vi "UpdateSetTerm.vi"(2 "State In":T1 {"BlockNodeState"."Draw Style" items=["FunctionBlock", "ExpressVI", "Variable", "Elemental I/O", "32x32 Icon", "FunctionBlockCompact"]; "BlockNodeState"."Terminal Data"."Terminal Flags" format="%.0b"}) -> (0 "State Out":T1 {"BlockNodeState"."Draw Style" items=["FunctionBlock", "ExpressVI", "Variable", "Elemental I/O", "32x32 Icon", "FunctionBlockCompact"]; "BlockNodeState"."Terminal Data"."Terminal Flags" format="%.0b"})   [LabVIEW 2017, in "Set DDT Attributes.lvlib"]
uses:
  <vilib>/express/express signal manip/GetorSetDDTAttributes/Set DDT Attributes/Set DDT Attributes.lvlib
  <vilib>/express/express signal manip/GetorSetDDTAttributes/Set DDT Attributes/State.ctl
  <vilib>/BlockNodeSupport/BlockNodeState.ctl
  <vilib>/BlockNodeSupport/TerminalData.ctl
  <vilib>/picture/picture.llb/imagedata.ctl
  <vilib>/express/express signal manip/GetorSetDDTAttributes/Shared VIs/Attributes data.ctl
  <vilib>/express/express signal manip/GetorSetDDTAttributes/Shared VIs/Input.ctl
  <vilib>/express/express signal manip/GetorSetDDTAttributes/Shared VIs/Attributes name.ctl
  <vilib>/express/express signal manip/GetorSetDDTAttributes/Shared VIs/GetSetShared.lvlib
  <vilib>/express/express signal manip/GetorSetDDTAttributes/Set DDT Attributes/Set DDT Properties.xnode
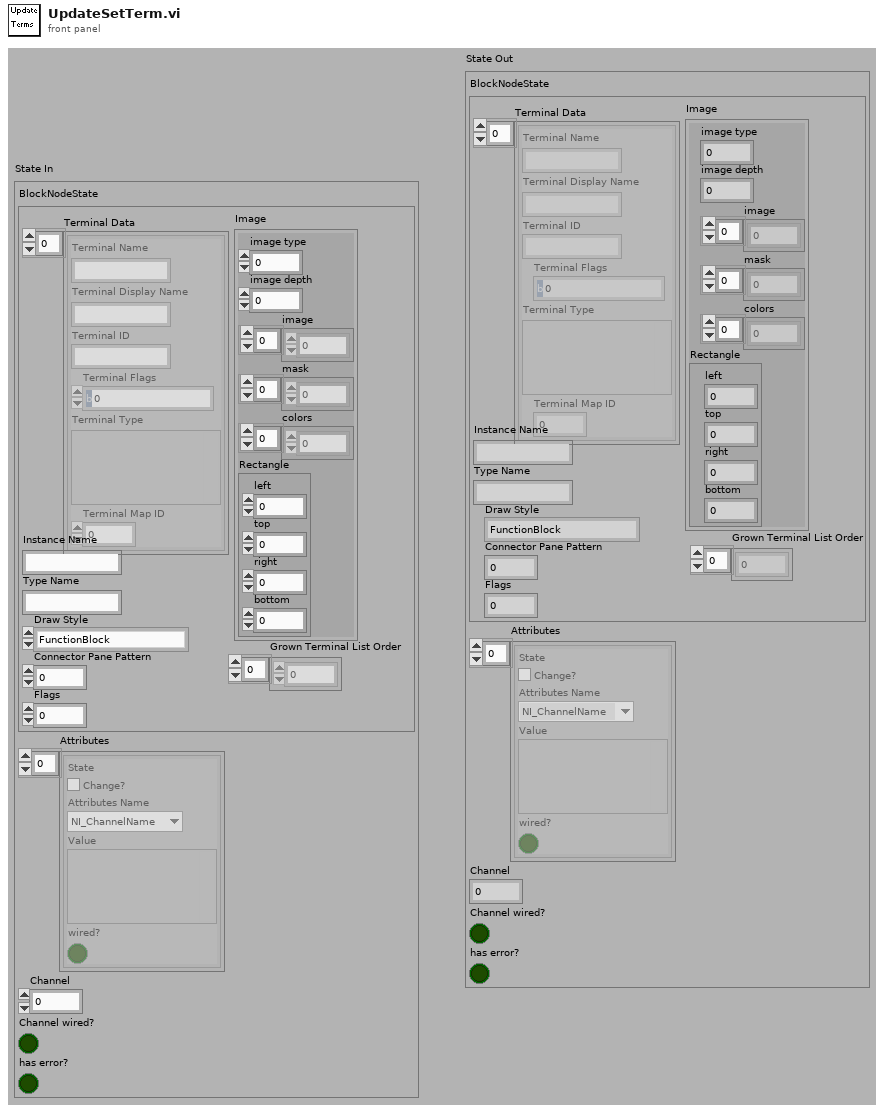
[diagram p1: front panel]
types:
  T1 = typedef "Set DDT Attributes.lvlib/Set DDT Properties.xnode/State.ctl" = cluster{"BlockNodeState":T2, "Attributes":T5[], "Channel":u32, "Channel wired?":bool, "has error?":bool}
  T2 = typedef "BlockNodeState.ctl" = cluster{"Terminal Data":T3[], "Instance Name":string, "Type Name":string, "Draw Style":i32, "Connector Pane Pattern":i32, "Flags":i32, "Grown Terminal List Order":i32[], "Image":T4}
  T3 = typedef "TerminalData.ctl" = cluster{"Terminal Name":string, "Terminal Display Name":string, "Terminal ID":string, "Terminal Flags":i32, "Terminal Type":variant, "Terminal Map ID":i32}
  T4 = typedef "imagedata.ctl" = cluster{"image type":i32, "image depth":i32, "image":u8[], "mask":u8[], "colors":u32[], "Rectangle":cluster{"left":i16, "top":i16, "right":i16, "bottom":i16}}
  T5 = typedef "GetSetShared.lvlib/Attributes data.ctl" = cluster{"State":T6, "Attributes Name":T7, "Value":variant, "wired?":bool}
  T6 = typedef "GetSetShared.lvlib/Input.ctl" = bool
  T7 = typedef "GetSetShared.lvlib/Attributes name.ctl" = enum16{"NI_ChannelName", "NI_ExpIsRelativeTime", "NI_ExpTimeStamp", "NI_ExpStartTimeStamp", "NI_ExpXDimension", "NI_UnitDescription"}
  T8 = cluster{"Terminal Name":string, "Terminal Display Name":string, "Terminal ID":string, "Terminal Flags":i32, "Terminal Type":variant, "Terminal Map ID":i32}
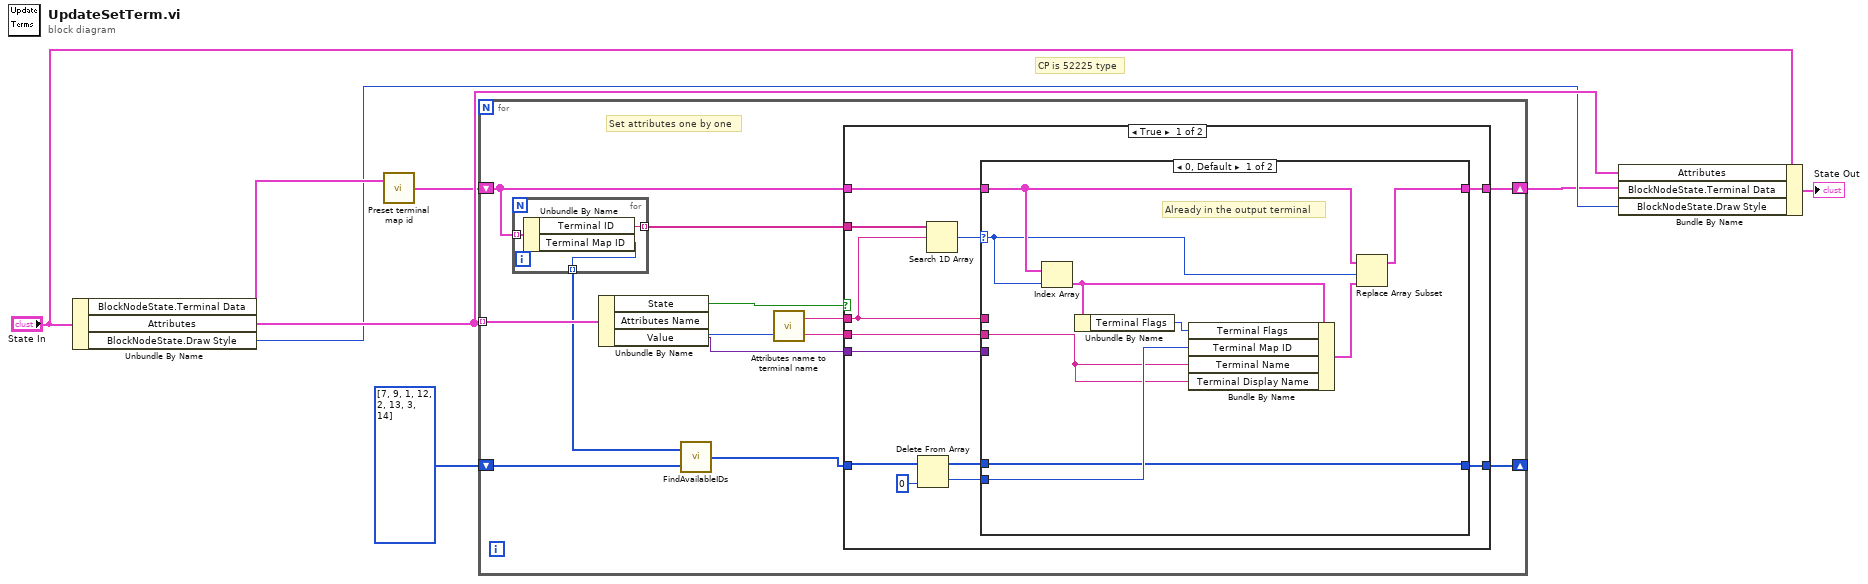
[diagram p0: block diagram]
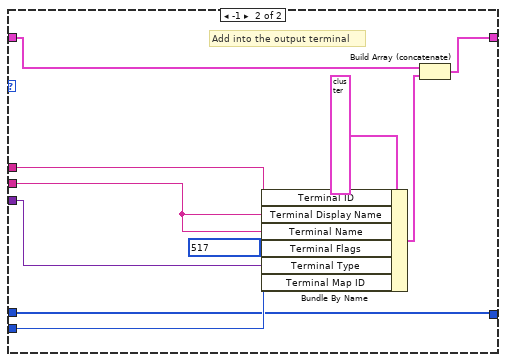
[diagram p2: hidden frame]
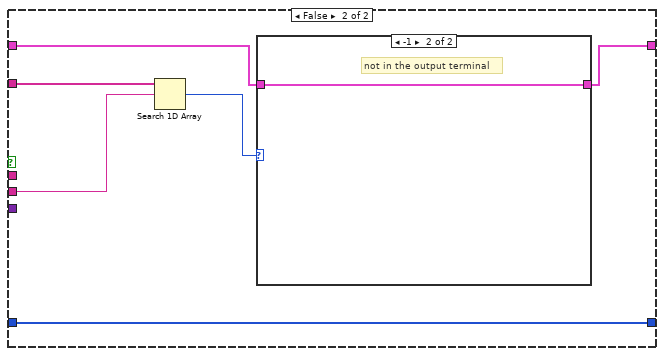
[diagram p3: hidden frame]
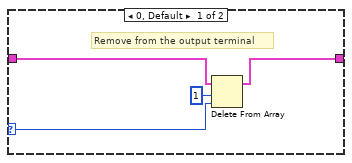
[diagram p4: hidden frame]
diagram:
  # "CP is 52225 type"
  n1 = Unbundle By Name("State In") -> ("BlockNodeState.Terminal Data"=w7:T3[], "Attributes"=w8:T5[], "BlockNodeState.Draw Style"=w6:i32)
  n2 = call <vilib>:"Preset terminal map id.vi"("Terminal Data in"=w7) -> ("Terminal Data out"=w2:T3[])  [unwired: 1 in]
  n3 = for {
    tunnel: w8 -> [w21] mode=indexing
    shift-right: [w20] -> w3
    shift-left: w2 -> [w19]
    shift-right: [w15] -> _
    shift-left: i32[] [7, 9, 1, 12, 2, 13, 3, 14] ("available map id") -> [w13]
    # "Set attributes one by one"
    n4 = for {
      tunnel: w19 -> [w24] mode=indexing
      tunnel: [w23] -> w14 mode=indexing
      tunnel: [w22] -> w11 mode=indexing
      n5 = Unbundle By Name(w24) -> ("Terminal ID"=w23:string, "Terminal Map ID"=w22:i32)
    }
    n6 = Unbundle By Name(w21) -> ("State"=w10:T6, "Attributes Name"=w18:T7, "Value"=w16:variant)
    n7 = call <vilib>:"FindAvailableIDs.vi"("All ids"=w13, "Unavailable ids"=w11) -> ("available map id"=w12:i32[])
    n8 = call <vilib>:"Attributes name to terminal name.vi"("Attributes Name"=w18) -> ("terminal Name"=w17:string, "Terminal ID"=w9:string)  [unwired: 1 out]
    n9 = case shown="True" w10 {
      tunnel: w19 -> [w35 w58]
      tunnel: [w34 w57] -> w20
      tunnel: w14 -> [w36 w61]
      tunnel: w17 -> [w31 w60]
      tunnel: w16 -> [w32 _]
      tunnel: w12 -> [w28 w56]
      tunnel: [w30 w56] -> w15
      tunnel: w9 -> [w25 _]
      frame True {
        n10 = Delete From Array(array=w28, index=0) -> (deleted portion=w29:i32, array with subset deleted=w26:i32[])  [unwired: 1 in]
        n11 = Search 1D Array(1D array=w36, element=w25) -> (index of element=w33:i32)  [unwired: 1 out]
        n12 = case shown="0, Default" w33 {
          selector: w33 -> [w43 _]
          tunnel: w35 -> [w44 w52]
          tunnel: [w41 w51] -> w34
          tunnel: w32 -> [_ w47]
          tunnel: w31 -> [w38 w50]
          tunnel: w29 -> [w45 w49]
          tunnel: [w40 w48] -> w30
          tunnel: w26 -> [w40 w48]
          tunnel: w25 -> [_ w46]
          frame 0, Default {
            # "Already in the output terminal"
            n13 = Index Array(array=w44, index=w43) -> (element=w39:T3)
            n14 = Unbundle By Name(w39) -> ("Terminal Flags"=w37:i32)
            n15 = Bundle By Name(cluster=w39, "Terminal Flags"=w37, "Terminal Map ID"=w45, "Terminal Name"=w38, "Terminal Display Name"=w38) -> (w42:T3)
            n16 = Replace Array Subset(array=w44, new element=w42, index=w43) -> (w41:T3[])
          }
          frame -1 {
            # "Add into the output terminal"
            n17 = Bundle By Name(cluster=T8 {"Terminal Name"="", "Terminal Display Name"="", "Terminal ID"="", "Terminal Flags"=0, "Terminal Type"=variant, "Terminal Map ID"=0} ("XNTerminalData"), "Terminal ID"=w46, "Terminal Display Name"=w50, "Terminal Name"=w50, "Terminal Flags"=517, "Terminal Type"=w47, "Terminal Map ID"=w49) -> (w53:T8)
            n18 = Build Array (concatenate)(w52, w53) -> (w51:T3[])
          }
        }
      }
      frame False {
        n19 = Search 1D Array(1D array=w61, element=w60) -> (index of element=w59:i32)  [unwired: 1 out]
        n20 = case shown="-1" w59 {
          selector: w59 -> [w64 _]
          tunnel: [w62 w66] -> w57
          tunnel: w58 -> [w65 w66]
          frame 0, Default {
            # "Remove from the output terminal"
            n21 = Delete From Array(array=w65, length=1, index=w64) -> (array with subset deleted=w62:T3[])  [unwired: 1 out]
          }
          frame -1 {
            # "not in the output terminal"
          }
        }
      }
    }
  }
  n22 = Bundle By Name(cluster="State In", "Attributes"=w8, "BlockNodeState.Terminal Data"=w3, "BlockNodeState.Draw Style"=w6) -> (→"State Out":T1)
